vi "XNET Write (Frame Ethernet).vi"(0 "session in":refnum<k21>, 5 "data":T1[](array[typedef]) {"fcs" format="%08x"; "network timestamp" format="%<%.7X\n%x>T"; "frame data" format="%x"; "local timestamp" format="%<%.7X\n%x>T"; "type" items=["Ethernet Data"=0, "Delay"=225, "Future Time Wait"=226]}, 9 "timeout (10)":dbl=10.0 format="%.2g", 11 "error in (no error)":errorcluster) -> (4 "session out":refnum<k21>, 15 "error out":errorcluster)   [LabVIEW 2018]
doc: "Writes data to a session as an array of Ethernet frames. The session must use an Ethernet interface and a mode of Frame Output Stream."
uses:
  XNET Frame Ethernet.ctl
  XNET Frame Type Ethernet.ctl
  nixlvapi.dll
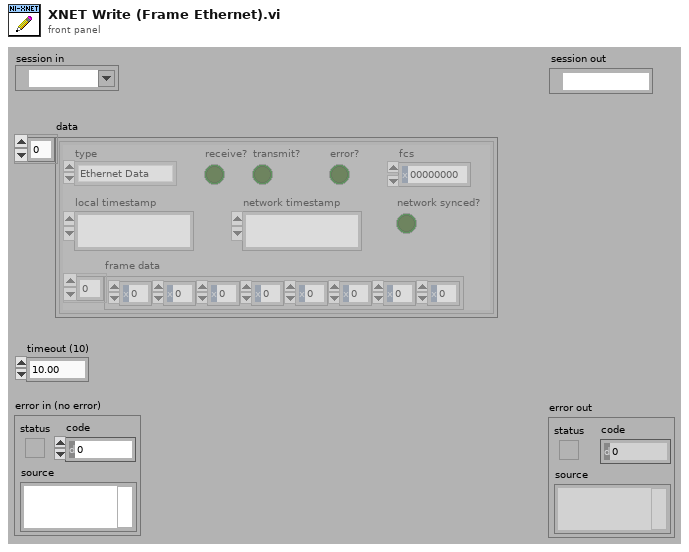
[diagram p1: front panel]
types:
  T1 = typedef "XNET Frame Ethernet.ctl" = cluster{"local timestamp":timestamp, "network timestamp":timestamp, "frame data":u8[], "fcs":u32, "type":T2, "network synced?":bool, "receive?":bool, "transmit?":bool, "error?":bool}
  T2 = typedef "XNET Frame Type Ethernet.ctl" = u16
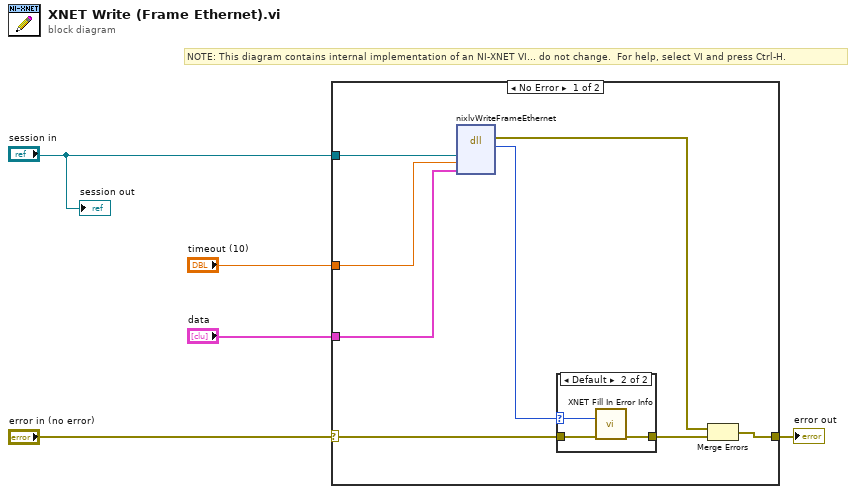
[diagram p0: block diagram]
diagram:
  # "NOTE: This diagram contains internal implementation of an NI-XNET VI... do not change.  For help, select VI and press Ctrl-H."
  n1 = case shown="No Error" "error in (no error)" {
    selector: "error in (no error)" -> [w12 w18]
    tunnel: "session in" -> [w13 _]
    tunnel: [w8 w18] -> w5
    tunnel: "timeout (10)" -> [w9 _]
    tunnel: "data" -> [w6 _]
    frame No Error {
      n2 = dll-call lib="nixlvapi.*" fn="nixlvWriteFrameEthernet"("SessionRef"=w13, "Timeout"=w9, "Data"=w6) -> (error out=w7:errorcluster, "return type"=w10:i32)  [unwired: 5 in, 2 out]
      n3 = case shown="Default" w10 {
        selector: w10 -> [_ w15]
        tunnel: w12 -> [w14 w16]
        tunnel: [w14 w17] -> w11
        frame 0 {
        }
        frame Default {
          n4 = call "XNET Fill In Error Info.vi"("status code"=w15, "error in"=w16) -> ("error out"=w17:errorcluster)  [unwired: 13 out]
        }
      }
      n5 = Merge Errors(w7, w11) -> (w8:errorcluster)
    }
    frame Error {
    }
  }
  "error out" <- w5
  "session out" <- "session in"
